vi "Preview_Error.vi"(8 "error in (no error)":errorcluster, 10 "IB_Tree.lvclass":refnum<class "IB_Tree.lvclass">, 11 "IB_Tree_Item_Proj_Container in":refnum<class "IB_Tree_Item_Proj_Container.lvclass">) -> (0 "error out":errorcluster, 3 "IB_Tree_Item_Proj_Container out":refnum<class "IB_Tree_Item_Proj_Container.lvclass">)   [LabVIEW 2020, in "IB_Tree_Item_Proj_Container.lvclass"]
uses:
  <vilib>/AppBuilder/IB_Classes/Tree_Item_Proj_Container/IB_Tree_Item_Proj_Container.lvclass
  <vilib>/AppBuilder/IB_Classes/Tree_Item_Proj_Container/IB_Tree_Item_Proj_Container.lvclass/IB_Tree_Item_Proj_Container.ctl
  <resource>/Framework/Providers/Builds/Installer/CDK_GLOBAL_STRINGS.vi
  <vilib>/AppBuilder/IB_Classes/Tree_Item/IB_Tree_Item.lvclass
  <vilib>/AppBuilder/IB_Classes/Tree/IB_Tree.lvclass
  e:/builds/penguin/labview/branches/2020/dev/dist/vi.lib/AppBuilder/IB_Classes/Tree_Item_Proj/IB_Tree_Item_Proj.lvclass
  e:/builds/penguin/labview/branches/2020/dev/dist/vi.lib/AppBuilder/IB_Classes/Tree_Item/IB_Tree_Item.lvclass
  e:/builds/penguin/labview/branches/2020/dev/dist/vi.lib/AppBuilder/IB_Classes/Tree_Item_Proj_Container/IB_Tree_Item_Proj_Container.lvclass
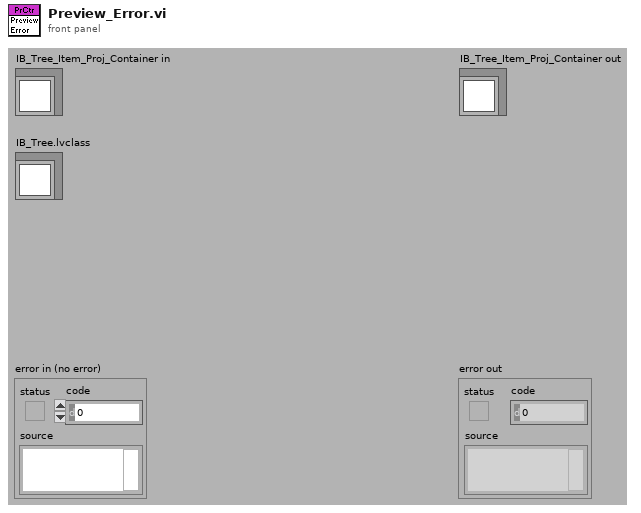
[diagram p1: front panel]
types:
  T1 = typedef "IB_Tree_Item.ctl" = cluster{"symbol index":i32, "child tag":string, "parentTag":string, "left cell name":string}
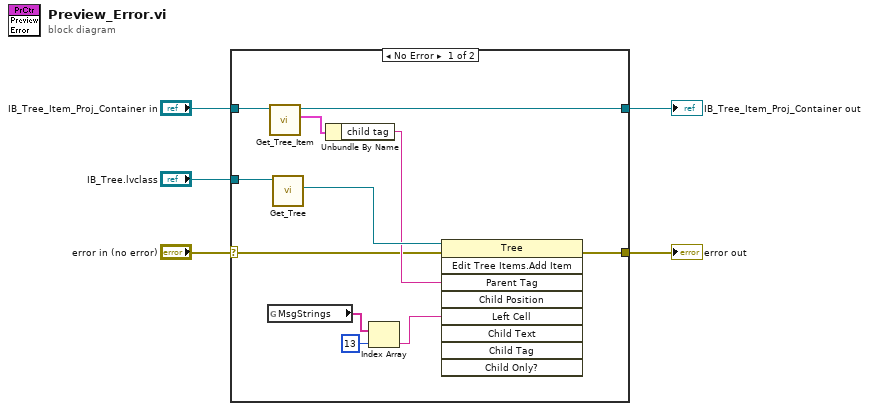
[diagram p0: block diagram]
diagram:
  n1 = case shown="No Error" "error in (no error)" {
    selector: "error in (no error)" -> [w7 w18]
    tunnel: [w6 w18] -> w4
    tunnel: [w12 w17] -> w2
    tunnel: "IB_Tree_Item_Proj_Container in" -> [w13 w17]
    tunnel: "IB_Tree.lvclass" -> [w11 _]
    frame No Error {
      n2 = global read "CDK_GLOBAL_STRINGS.vi" "MsgStrings"() -> (w16:string[])
      n3 = call <vilib>:"Get_Tree_Item.vi"("IB_TreeItem in"=w13) -> ("data"=w14:T1, "IB_TreeItem out"=w12:refnum<class "IB_Tree_Item_Proj_Container.lvclass">)  [unwired: 1 in, 8 out]
      n4 = call <vilib>:"Get_Tree.vi"("IB_Tree in"=w11) -> ("ctl"=w10:refnum<vi>)  [unwired: 1 in, 9 out]
      n5 = Unbundle By Name(w14) -> ("child tag"=w8:string)
      n6 = Index Array(array=w16, index=13) -> (element=w9:string)
      n7 = invoke class="Tree" method="Edit Tree Items.Add Item"(reference=w10, error in=w7, "Parent Tag"=w8, "Left Cell"=w9) -> (error out=w6:errorcluster)  [unwired: 5 in, 8 out]
    }
    frame Error {
    }
  }
  "error out" <- w4
  "IB_Tree_Item_Proj_Container out" <- w2
